vi "Stream Basic with Stream-Out.vi"() -> ()   [LabVIEW 2020]
uses:
  <vilib>/measure/NI_MABase.lvlib
panel:
  out "Desired #Updates":dbl
  out "Actual #Updates":u32
  in  "Update Stream-Out":bool
  in  "Function":u16(ring) items=["Sine Wave", "Triangle Wave", "Square Wave", "Sawtooth Wave"]
  in  "Offset":dbl=2.0 format="%.3g"
  in  "Amplitude (Peak-to-Peak)":dbl=4.0 format="%.3g"
  in  "Frequency":dbl=10.0 format="%.3f"
  in  "#Seconds on Graph":dbl=1.0 format="%.2f"
  out "SampleRate (Hz)":dbl format="%.3f"
  out "NumReadAddresses":i32
  in  "STREAM_RESOLUTION_INDEX":i32
  in  "STREAM_SETTLING_US":i32
  in  "AIN_ALL_RANGE":dbl=10.0 format="%.3f"
  out "ScansPerRead":i32
  out "ConnectionType Out":i32
  out "DeviceType Out":i32
  in  "Identifier":string="LJM_idANY"
  in  "ConnectionType":string="LJM_ctANY"
  in  "DeviceType":string="LJM_dtANY"
  out "DeviceScanBacklog":i32
  out "LJMScanBacklog":i32
  out "Data":dbl[][](array[numeric]) format="%.3f"
  out "Waveform Graph":dbl[][](graph)
  in  "Scan List":string[](array[string])=["AIN0", "STREAM_OUT0"]
  out "# of iterations":i32
  in  "Scan Rate (Hz)":dbl=100.0 format="%.3f"
  in  "stop":bool
  out "Error Message":string
  # "Stream-Out settings for DAC0."
  # "To remove an element, right-click\non it, select Data Operations =>\nRemove Element.\n\nTo empty an array, right-click\nnear the edge, select Data\nOperations => Empty Array.\n\nOther useful operations:  From the\nOperate menu are \"Make Current\nValues Default\" and \"Reinitialize\nTo Default\"."
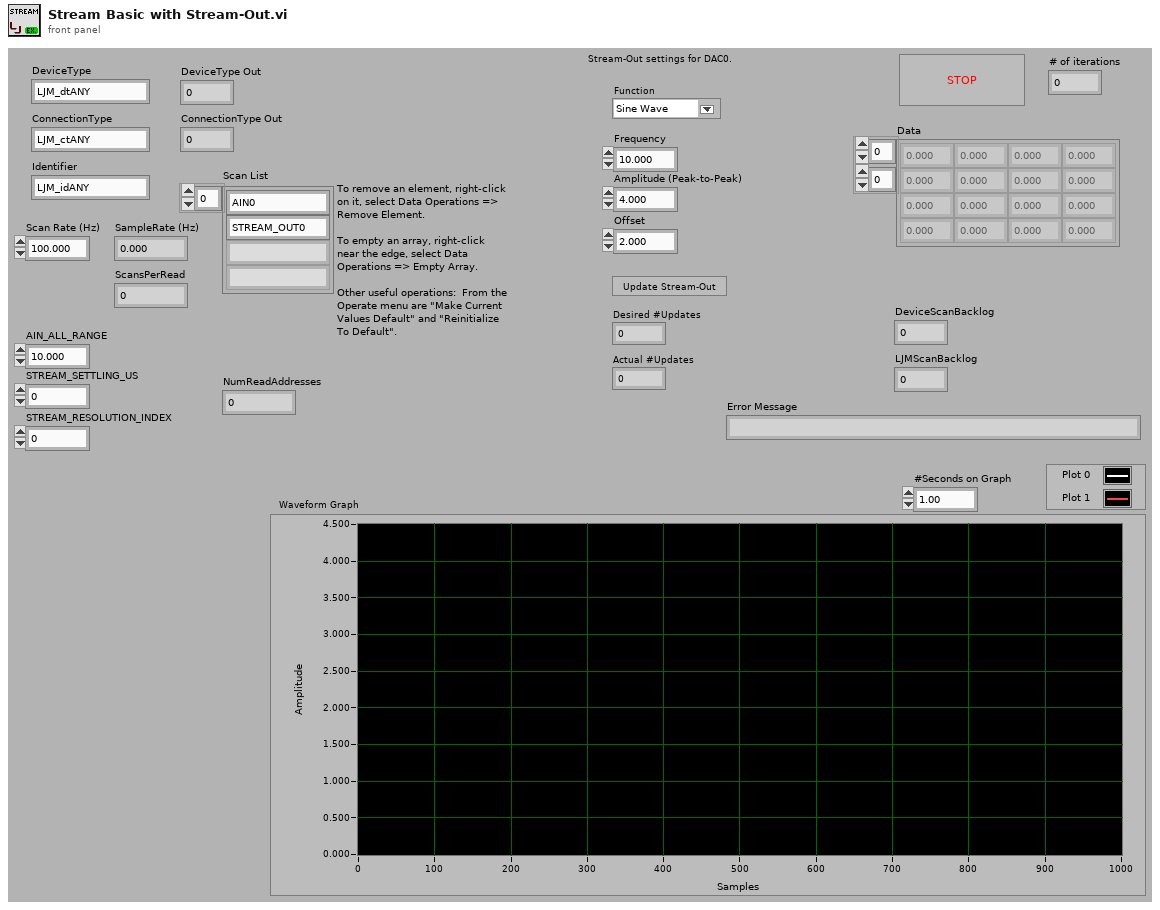
[diagram p1: front panel]
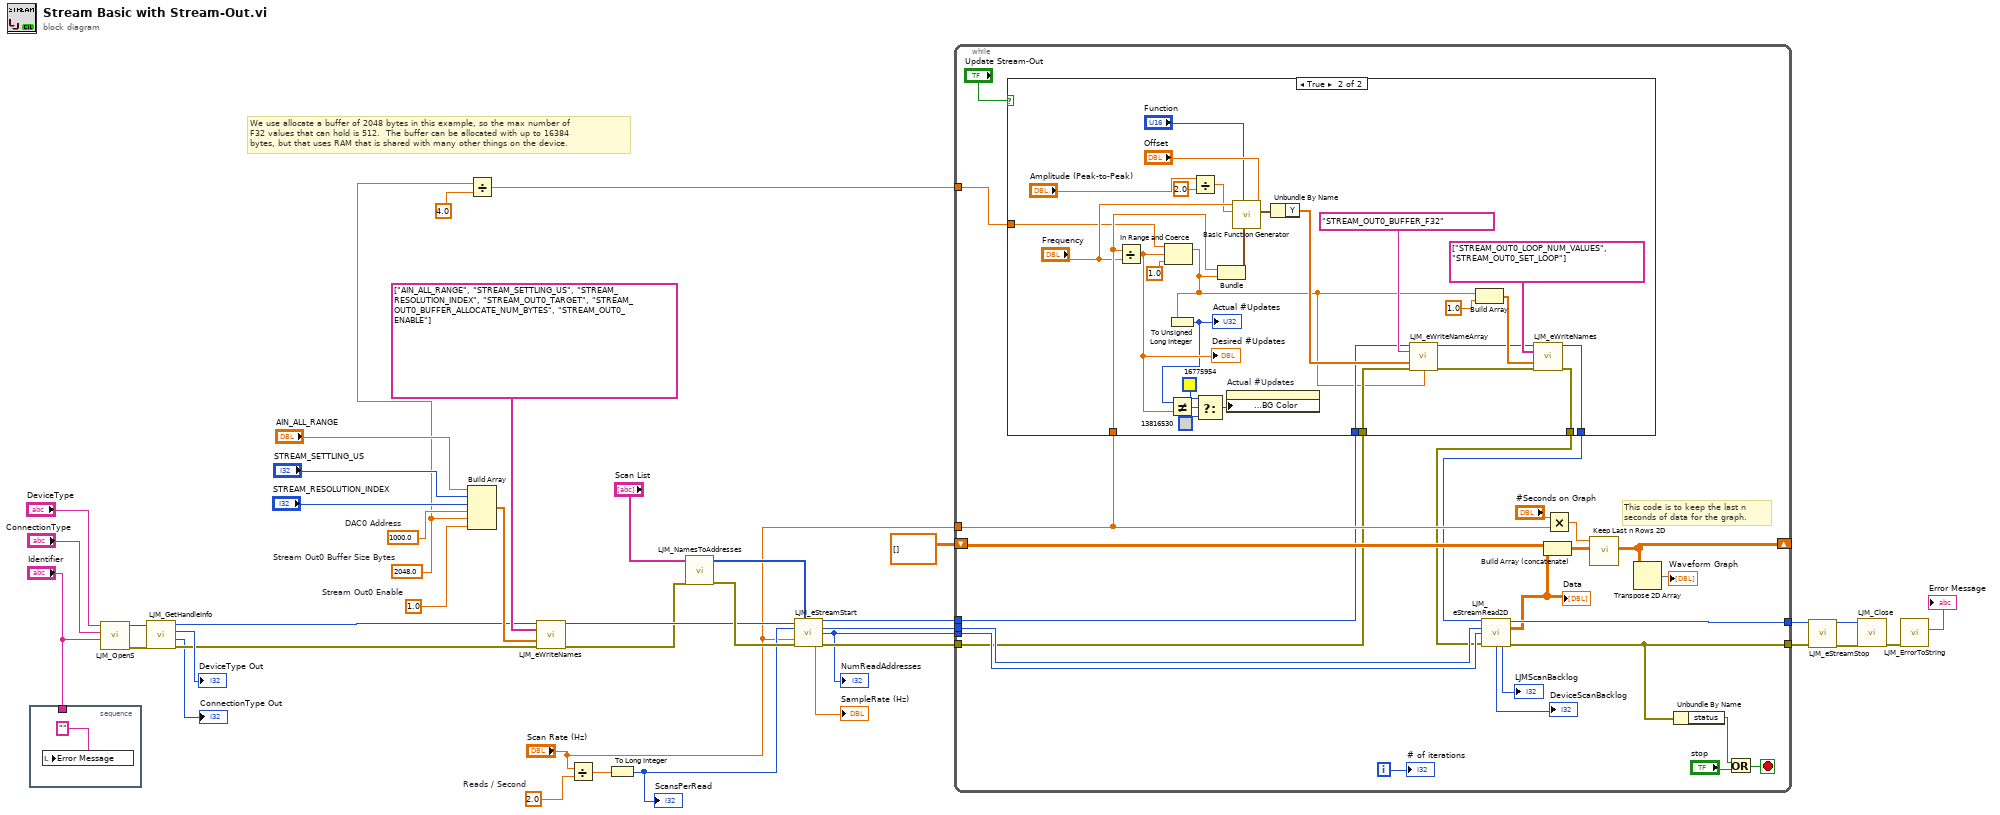
[diagram p0: block diagram]
diagram:
  w5 = 1.0  # Stream Out0 Enable
  w2 = 2048.0  # Stream Out0 Buffer Size Bytes
  w6 = 1000.0  # DAC0 Address
  w25 = 2.0  # Reads / Second
  # "We use allocate a buffer of 2048 bytes in this example, so the max number of\nF32 values that can hold is 512.  The buffer can be allocated with up to 16384\nbytes, but that uses RAM that is shared with many other things on the device."
  n1 = stacked-sequence {
    tunnel: "Identifier" -> [_]
    frame #0 {
      n2 = local write "Error Message"("" ("Error Message")) -> ()
    }
  }
  n3 = call "LJM_OpenS.vi"("Identifier"="Identifier", "ConnectionType"="ConnectionType", "DeviceType"="DeviceType") -> ("error out"=w32:errorcluster, "Handle"=w29:i32)  [unwired: 7 in]
  n4 = call "LJM_GetHandleInfo.vi"("error in"=w32, "Handle In"=w29) -> ("error out"=w7:errorcluster, "ConnectionType"=→"ConnectionType Out":i32, "DeviceType"=→"DeviceType Out":i32, "Handle Out"=w8:i32)  [unwired: 2 in, 4 out]
  n5 = Divide(x=w2, y=4.0 ("upper limit")) -> (x/y=w1:dbl)
  n6 = Build Array("AIN_ALL_RANGE", "STREAM_SETTLING_US", "STREAM_RESOLUTION_INDEX", w6, w2, w5) -> (w18:dbl[])
  n7 = call "LJM_eWriteNames.vi"("Handle In"=w8, "aNames"=string[] ["AIN_ALL_RANGE", "STREAM_SETTLING_US", "STREAM_RESOLUTION_INDEX", "STREAM_OUT0_TARGET", "STREAM_OUT0_BUFFER_ALLOCATE_NUM_BYTES", "STREAM_OUT0_ENABLE"], "aValuesIn"=w18, "error in"=w7) -> ("Handle Out"=w22:i32, "error out"=w21:errorcluster)  [unwired: 9 in, 1 out]
  n8 = Divide(x="Scan Rate (Hz)", y=w25) -> (x/y=w24:dbl)
  n9 = To Long Integer(number=w24) -> (32bit integer=w23:i32)
  "ScansPerRead" <- w23
  n10 = call "LJM_NamesToAddresses.vi"("error in"=w21, "aNames"="Scan List") -> ("error out"=w26:errorcluster, "aAddresses"=w15:i32[])  [unwired: 7 in, 1 out]
  n11 = call "LJM_eStreamStart.vi"("Handle In"=w22, "aScanList"=w15, "ScansPerRead"=w23, "ScanRate"="Scan Rate (Hz)", "error in"=w26) -> ("Handle Out"=w39:i32, "ScansPerRead Out"=w11:i32, "NumReadAddresses"=w13:i32, "Actual SampleRate"=→"SampleRate (Hz)":dbl, "error out"=w40:errorcluster)  [unwired: 5 in, 1 out]
  "NumReadAddresses" <- w13
  n12 = while {
    tunnel: [w61] -> w37
    tunnel: w39 -> [w46]
    tunnel: w13 -> [w50]
    tunnel: w11 -> [w49]
    shift-right: [w51] -> _
    shift-left: dbl[][] [] -> [w55]
    tunnel: "Scan Rate (Hz)" -> [w48]
    tunnel: w1 -> [w42]
    tunnel: w40 -> [w45]
    tunnel: [w58] -> w38
    i -> [w62]
    stop <- w63 stop-if-true
    # "This code is to keep the last n\nseconds of data for the graph."
    n13 = case shown="True" "Update Stream-Out" {
      tunnel: w48 -> [_ w93]
      tunnel: w46 -> [w66 w82]
      tunnel: w45 -> [w67 w81]
      tunnel: [w67 w80] -> w44
      tunnel: [w66 w79] -> w43
      tunnel: w42 -> [_ w78]
      frame False {
      }
      frame True {
        n14 = Divide(x=w93, y="Frequency") -> (x/y=w70:dbl)
        "Desired #Updates" <- w70
        n15 = In Range and Coerce(upper limit=w78, x=w70, lower limit=1.0) -> (coerced(x)=w69:dbl)  [unwired: 1 out]
        n16 = To Unsigned Long Integer(number=w69) -> (unsigned 32bit integer=w68:u32)
        "Actual #Updates" <- w68
        n17 = Not Equal?(x=w68, y=w70) -> (x != y?=w73:bool)
        n18 = Divide(x="Amplitude (Peak-to-Peak)", y=2.0) -> (x/y=w75:dbl)
        n19 = Select(t=u32 16775954, s=w73, f=u32 13816530) -> (s? t:f=w74:u32)
        n20 = Bundle("Scan Rate (Hz)"=w93, "lower limit"=w69) -> (w95:cluster{"Scan Rate (Hz)":dbl, "lower limit":dbl})  [unwired: 1 in]
        n21 = property on="Actual #Updates" class="DigNum (strict)"("Numeric Text.Text Colors:BG Color"=w74) -> ()  [unwired: 2 in, 2 out]
        n22 = call <vilib>:"Basic Function Generator.vi"("offset"="Offset", "sampling info"=w95, "signal type"="Function", "amplitude"=w75, "frequency"="Frequency") -> ("signal out"=w94:waveform(dbl))  [unwired: 4 in, 2 out]
        n23 = Unbundle By Name(w94) -> ("Y"=w83:dbl[])
        n24 = call "LJM_eWriteNameArray.vi"("Handle In"=w82, "Name"="STREAM_OUT0_BUFFER_F32" ("String"), "aValues"=w83, "error in"=w81, "NumValues"=w69) -> ("Handle Out"=w86:i32, "error out"=w85:errorcluster)  [unwired: 8 in, 1 out]
        n25 = Build Array(w69, 1.0 ("element")) -> (w87:dbl[])
        n26 = call "LJM_eWriteNames.vi"("Handle In"=w86, "aNames"=string[] ["STREAM_OUT0_LOOP_NUM_VALUES", "STREAM_OUT0_SET_LOOP"], "aValuesIn"=w87, "error in"=w85) -> ("Handle Out"=w79:i32, "error out"=w80:errorcluster)  [unwired: 9 in, 1 out]
      }
    }
    n27 = call "LJM_eStreamRead2D.vi"("Handle In"=w43, "ScansPerRead"=w49, "NumAddresses"=w50, "error in"=w44) -> ("Handle Out"=w61:i32, "aData Out"=w56:dbl[][], "DeviceScanBacklog"=→"DeviceScanBacklog":i32, "LJMScanBacklog"=→"LJMScanBacklog":i32, "error out"=w58:errorcluster)  [unwired: 7 in]
    "Data" <- w56
    n28 = Build Array (concatenate)(w55, w56) -> (w53:dbl[][])
    n29 = Multiply(x="#Seconds on Graph", y=w48) -> (x*y=w52:dbl)
    n30 = call "Keep Last n Rows 2D.vi"("Array"=w53, "# Rows to Keep"=w52) -> ("Last n Rows"=w51:dbl[][])  [unwired: 9 in]
    n31 = Transpose 2D Array(2D array=w51) -> (transposed array=→"Waveform Graph":dbl[][])
    n32 = Unbundle By Name(w58) -> ("status"=w64:bool)
    n33 = Or(x=w64, y="stop") -> (x .or. y?=w63:bool)
    "# of iterations" <- w62
  }
  n34 = call "LJM_eStreamStop.vi"("Handle In"=w37, "error in"=w38) -> ("Handle Out"=w35:i32, "error out"=w36:errorcluster)  [unwired: 12 in]
  n35 = call "LJM_Close.vi"("error in"=w36, "Handle"=w35) -> ("error out"=w34:errorcluster)  [unwired: 9 in]
  n36 = call "LJM_ErrorToString.vi"("error in"=w34) -> ("String"=→"Error Message":string)  [unwired: 10 in]
